vi "MAS.vi"(0 "System no.":i32=1 min=1 max=4 step=1, 2 "Slave axis":string[](array[string]), 3 "Master axis":string[](array[string]), 5 "error in":errorcluster) -> (19 "error out":errorcluster)   [LabVIEW 2020]
doc: "Set master axis."
panel:
  # "Set master axis."
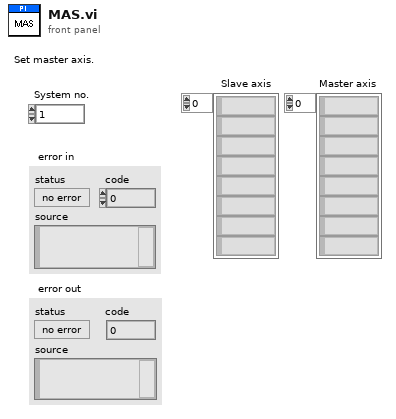
[diagram p1: front panel]
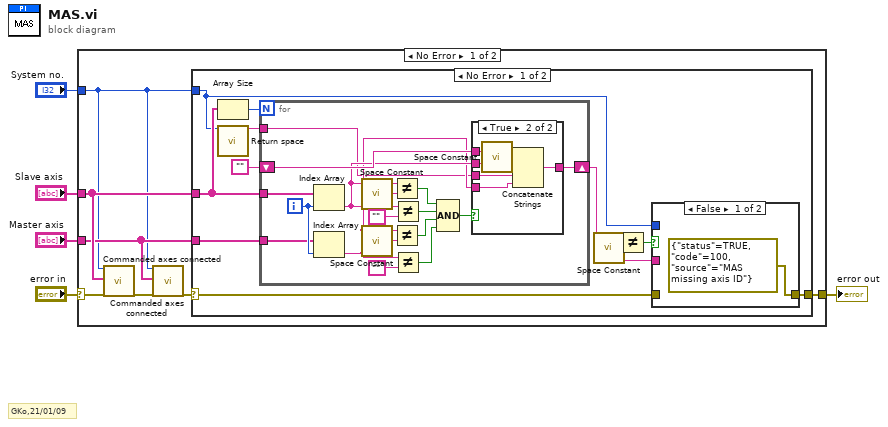
[diagram p0: block diagram]
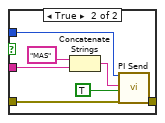
[diagram p2: hidden frame]
diagram:
  # "GKo,21/01/09"
  n1 = case shown="No Error" "error in" {
    selector: "error in" -> [w7 w57]
    tunnel: "Slave axis" -> [w12 _]
    tunnel: [w11 w57] -> w4
    tunnel: "Master axis" -> [w10 _]
    tunnel: "System no." -> [w9 _]
    frame No Error {
      n2 = call "Commanded axes connected.vi"("System no."=w9, "Commanded axes"=w12, "error in"=w7) -> ("error out"=w8:errorcluster)  [unwired: 16 out]
      n3 = call "Commanded axes connected.vi"("System no."=w9, "Commanded axes"=w10, "error in"=w8) -> ("error out"=w6:errorcluster)  [unwired: 16 out]
      n4 = case shown="No Error" w6 {
        selector: w6 -> [w13 w56]
        tunnel: w12 -> [w23 _]
        tunnel: [w18 w56] -> w11
        tunnel: w10 -> [w20 _]
        tunnel: w9 -> [w14 _]
        frame No Error {
          n5 = Array Size(array=w23) -> (size(s)=w16:i32)
          n6 = call "Return space.vi"("System no."=w14) -> ("String out"=w15:string)  [unwired: 1 in, 17 out]
          n7 = for {
            N: w16 -> [_]
            tunnel: w23 -> [w37]
            shift-right: [w46] -> w19
            shift-left: "" -> [w47]
            tunnel: w20 -> [w35]
            tunnel: w15 -> [w32]
            i -> [w36]
            n8 = Index Array(array=w37, index=w36) -> (element=w45:string)
            n9 = Index Array(array=w35, index=w36) -> (element=w34:string)
            n10 = call <vilib>:"Space Constant.vi"() -> ("String"=w48:string)
            n11 = call <vilib>:"Space Constant.vi"() -> ("String"=w43:string)
            n12 = Not Equal?(x=w45, y=w48) -> (x != y?=w41:bool)
            n13 = Not Equal?(x=w34, y=w43) -> (x != y?=w39:bool)
            n14 = Not Equal?(x=w45, y="") -> (x != y?=w40:bool)
            n15 = Not Equal?(x=w34, y="") -> (x != y?=w38:bool)
            n16 = Compound Arithmetic op=AND(w41, w40, w39, w38) -> (w33:bool)
            n17 = case shown="True" w33 {
              tunnel: w47 -> [w49 w55]
              tunnel: w45 -> [_ w52]
              tunnel: [w49 w54] -> w46
              tunnel: w34 -> [_ w51]
              tunnel: w32 -> [_ w50]
              frame False {
              }
              frame True {
                n18 = call <vilib>:"Space Constant.vi"() -> ("String"=w53:string)
                n19 = Concatenate Strings(w55, w53, w52, w50, w51) -> (w54:string)
              }
            }
          }
          n20 = call <vilib>:"Space Constant.vi"() -> ("String"=w21:string)
          n21 = Not Equal?(x=w19, y=w21) -> (x != y?=w17:bool)
          n22 = case shown="False" w17 {
            tunnel: w19 -> [_ w29]
            tunnel: w13 -> [_ w27]
            tunnel: w14 -> [_ w26]
            tunnel: [errorcluster {"status"=TRUE, "code"=100, "source"="MAS missing axis ID"} ("error out") w25] -> w18
            frame False {
            }
            frame True {
              n23 = Concatenate Strings("MAS", w29) -> (w28:string)
              n24 = call "PI Send.vi"("System no."=w26, "String to send"=w28, "Attach termination char.?"=TRUE ("Attach Linefeed?"), "error in"=w27) -> ("error out"=w25:errorcluster)  [unwired: 2 in, 13 out]
            }
          }
        }
        frame Error {
        }
      }
    }
    frame Error {
    }
  }
  "error out" <- w4
